vi "find circle corners - rescale back.vi"(5 "spot size":dbl, 7 "spot center":cdb, 11 "4 corners in":T1={"z (-pi/2)"=-1.0311345636926572+0.5736824521422934i, "z(inf)"=-0.5200164984937075+1.0975277942502903i, "z (pi/2)"=-1.0311345636926572+0.5736824521422934i, "z center"=-0.5136528600391839+0.580046090596817i, "z(0)"=-0.5200164984937075+1.0975277942502903i, "radius"=-1.0311345636926572}) -> (3 "4 corners out":T1={"z (-pi/2)"=-1.0311345636926572+0.5736824521422934i, "z(inf)"=-0.5200164984937075+1.0975277942502903i, "z (pi/2)"=-1.0311345636926572+0.5736824521422934i, "z center"=-0.5136528600391839+0.580046090596817i, "z(0)"=-0.5200164984937075+1.0975277942502903i, "radius"=-1.0311345636926572})   [LabVIEW 2021]
uses:
  circle corners.ctl
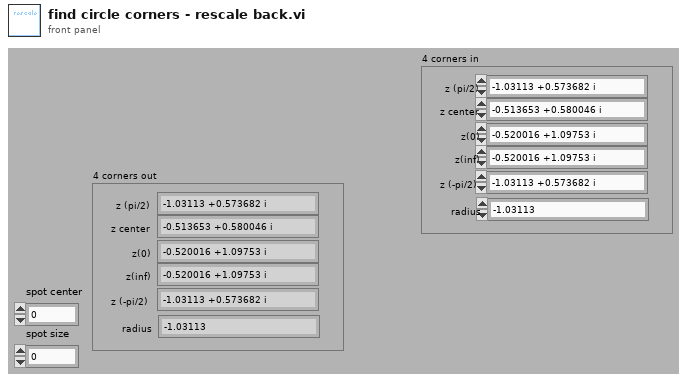
[diagram p1: front panel]
types:
  T1 = typedef "circle corners.ctl" = cluster{"z (-pi/2)":cdb, "z(inf)":cdb, "z (pi/2)":cdb, "z center":cdb, "z(0)":cdb, "radius":dbl}
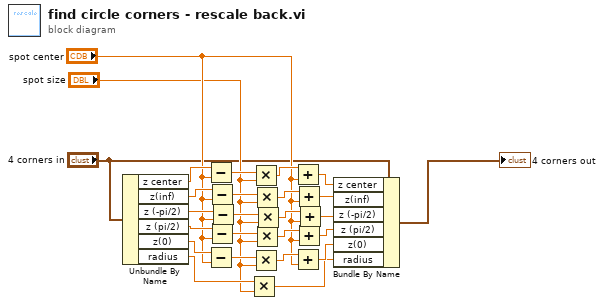
[diagram p0: block diagram]
diagram:
  n1 = Unbundle By Name("4 corners in") -> ("z center"=w25:cdb, "z(inf)"=w11:cdb, "z (-pi/2)"=w5:cdb, "z (pi/2)"=w16:cdb, "z(0)"=w15:cdb, "radius"=w7:dbl)
  n2 = Subtract(x=w25, y="spot center") -> (x-y=w26:cdb)
  n3 = Subtract(x=w15, y="spot center") -> (x-y=w18:cdb)
  n4 = Subtract(x=w11, y="spot center") -> (x-y=w12:cdb)
  n5 = Subtract(x=w16, y="spot center") -> (x-y=w20:cdb)
  n6 = Subtract(x=w5, y="spot center") -> (x-y=w23:cdb)
  n7 = Multiply(x=w7, y="spot size") -> (x*y=w6:dbl)
  n8 = Multiply(x=w26, y="spot size") -> (x*y=w24:cdb)
  n9 = Multiply(x=w18, y="spot size") -> (x*y=w17:cdb)
  n10 = Multiply(x=w12, y="spot size") -> (x*y=w10:cdb)
  n11 = Multiply(x=w20, y="spot size") -> (x*y=w19:cdb)
  n12 = Multiply(x=w23, y="spot size") -> (x*y=w22:cdb)
  n13 = Add(x=w24, y="spot center") -> (x+y=w21:cdb)
  n14 = Add(x=w17, y="spot center") -> (x+y=w14:cdb)
  n15 = Add(x=w10, y="spot center") -> (x+y=w9:cdb)
  n16 = Add(x=w19, y="spot center") -> (x+y=w13:cdb)
  n17 = Add(x=w22, y="spot center") -> (x+y=w8:cdb)
  n18 = Bundle By Name(cluster="4 corners in", "z center"=w21, "z(inf)"=w9, "z (-pi/2)"=w8, "z (pi/2)"=w13, "z(0)"=w14, "radius"=w6) -> (→"4 corners out":T1)
